vi "LDF Get Frame Publisher.vi"(9 "pPublisher":string, 10 "pFrameName":string, 11 "LDFHandle":u64) -> (1 "pPublisher out":string, 2 "pFrameName out":string, 3 "function return":i32)   [LabVIEW 2010, in "ldf_parser.lvlib"]
doc: "int WINAPI LDF_GetFramePublisher(long long LDFHandle, char* pFrameName, char* pPublisher);"
uses:
  ldf_parser.lvlib
  USB2XXX/trunk/USB2XXX/USB2XXX/vs2019/Release/USB2XXX.dll
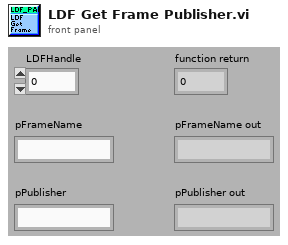
[diagram p1: front panel]
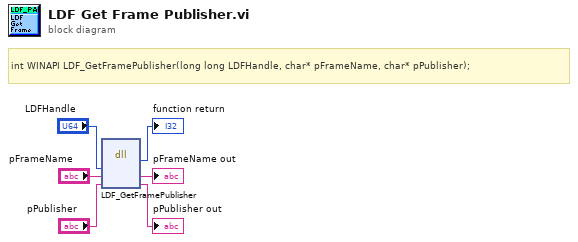
[diagram p0: block diagram]
diagram:
  # "int WINAPI LDF_GetFramePublisher(long long LDFHandle, char* pFrameName, char* pPublisher);"
  n1 = dll-call lib="E:/Projects/USB2XXX/trunk/USB2XXX/USB2XXX/vs2019/Release/USB2XXX.*" fn="LDF_GetFramePublisher"("LDFHandle"="LDFHandle", "pFrameName"="pFrameName", "pPublisher"="pPublisher") -> (→"function return":i32, "pFrameName"=→"pFrameName out":string, "pPublisher"=→"pPublisher out":string)  [unwired: 4 in, 2 out]
